vi "VI Tree.vi"   [LabVIEW 2015, in "IT8900A-E.lvlib"]
doc: "This is the instrument driver for the <INSTRUMENT NAME>. The VI Tree displays all the user-callable VIs of the instrument driver in an organized table."
uses:
  <instrlib>/IT8900/IT8900A-E.lvlib
panel:
  # "(c) 2014 <ITECH>.  ALL RIGHTS RESERVED."
  # "SEE DIAGRAM\nFOR VI TREE."
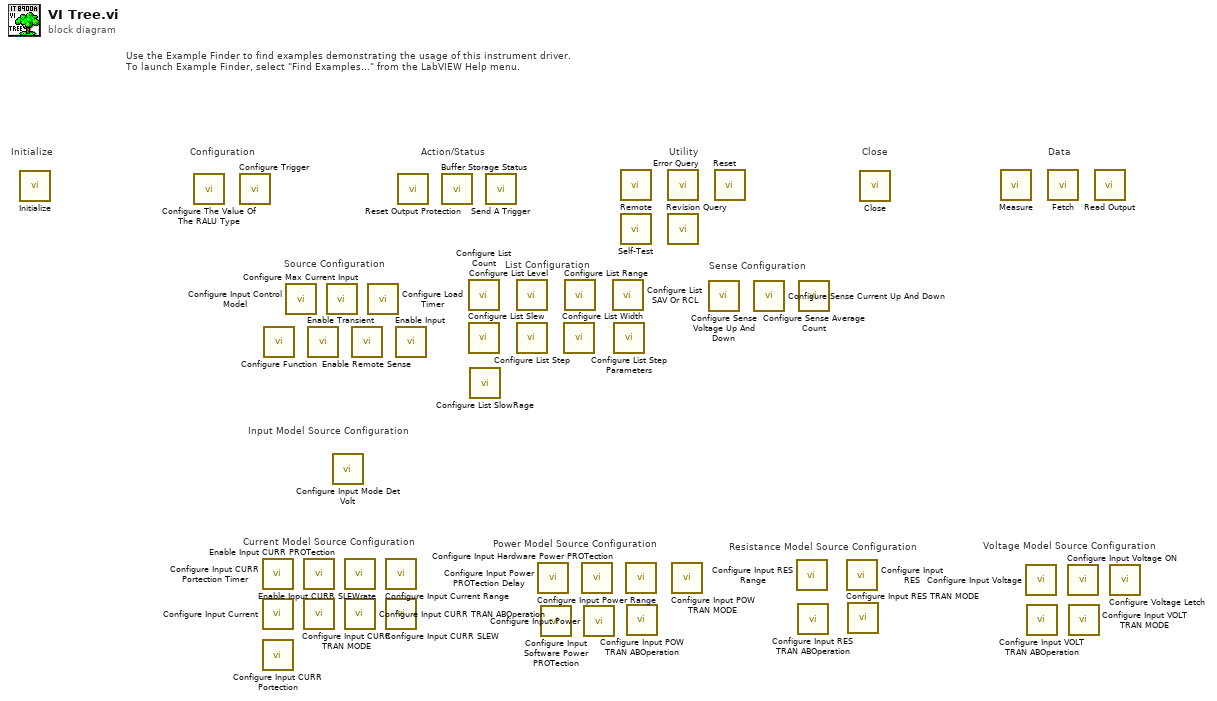
[diagram p0: block diagram]
diagram:
  # "Sense Configuration"
  # "List Configuration"
  # "Power Model Source Configuration"
  # "Resistance Model Source Configuration"
  # "Voltage Model Source Configuration"
  # "Current Model Source Configuration"
  # "Input Model Source Configuration"
  # "Source Configuration"
  # "Use the Example Finder to find examples demonstrating the usage of this instrument driver.\nTo launch Example Finder, select \"Find Examples...\" from the LabVIEW Help menu."
  # "Configuration"
  # "Utility"
  # "Data"
  # "Action/Status"
  # "Close"
  # "Initialize"
  n1 = call <instrlib>:"Initialize.vi"() -> ()  [unwired: 10 in, 2 out]
  n2 = call <instrlib>:"Configure The Value Of The RALU Type.vi"() -> ()  [unwired: 9 in, 2 out]
  n3 = call <instrlib>:"Configure Trigger.vi"() -> ()  [unwired: 10 in, 2 out]
  n4 = call <instrlib>:"Configure Input CURR Portection Timer.vi"() -> ()  [unwired: 10 in, 2 out]
  n5 = call <instrlib>:"Configure Input Current.vi"() -> ()  [unwired: 10 in, 2 out]
  n6 = call <instrlib>:"Configure Input CURR Portection.vi"() -> ()  [unwired: 10 in, 2 out]
  n7 = call <instrlib>:"Configure Function.vi"() -> ()  [unwired: 10 in, 2 out]
  n8 = call <instrlib>:"Configure Input Control Model.vi"() -> ()  [unwired: 10 in, 2 out]
  n9 = call <instrlib>:"Enable Input CURR PROTection.vi"() -> ()  [unwired: 10 in, 2 out]
  n10 = call <instrlib>:"Configure Input CURR TRAN MODE.vi"() -> ()  [unwired: 10 in, 2 out]
  n11 = call <instrlib>:"Enable Transient.vi"() -> ()  [unwired: 10 in, 2 out]
  n12 = call <instrlib>:"Configure Max Current Input.vi"() -> ()  [unwired: 10 in, 2 out]
  n13 = call <instrlib>:"Configure Input Mode Det Volt.vi"() -> ()  [unwired: 10 in, 2 out]
  n14 = call <instrlib>:"Enable Input CURR SLEWrate.vi"() -> ()  [unwired: 10 in, 2 out]
  n15 = call <instrlib>:"Configure Input CURR TRAN ABOperation.vi"() -> ()  [unwired: 10 in, 2 out]
  n16 = call <instrlib>:"Enable Remote Sense.vi"() -> ()  [unwired: 10 in, 2 out]
  n17 = call <instrlib>:"Configure Load Timer.vi"() -> ()  [unwired: 10 in, 2 out]
  n18 = call <instrlib>:"Configure Input Current Range.vi"() -> ()  [unwired: 10 in, 2 out]
  n19 = call <instrlib>:"Configure Input CURR SLEW.vi"() -> ()  [unwired: 10 in, 2 out]
  n20 = call <instrlib>:"Enable Input.vi"() -> ()  [unwired: 10 in, 2 out]
  n21 = call <instrlib>:"Reset Output Protection.vi"() -> ()  [unwired: 10 in, 2 out]
  n22 = call <instrlib>:"Buffer Storage Status.vi"() -> ()  [unwired: 7 in, 5 out]
  n23 = call <instrlib>:"Configure List Count.vi"() -> ()  [unwired: 10 in, 2 out]
  n24 = call <instrlib>:"Configure List Slew.vi"() -> ()  [unwired: 10 in, 2 out]
  n25 = call <instrlib>:"Configure List SlowRage.vi"() -> ()  [unwired: 10 in, 2 out]
  n26 = call <instrlib>:"Send A Trigger.vi"() -> ()  [unwired: 10 in, 2 out]
  n27 = call <instrlib>:"Configure List Level.vi"() -> ()  [unwired: 10 in, 2 out]
  n28 = call <instrlib>:"Configure List Step.vi"() -> ()  [unwired: 10 in, 2 out]
  n29 = call <instrlib>:"Configure Input Power PROTection Delay.vi"() -> ()  [unwired: 10 in, 2 out]
  n30 = call <instrlib>:"Configure Input Software Power PROTection.vi"() -> ()  [unwired: 10 in, 2 out]
  n31 = call <instrlib>:"Configure List Width.vi"() -> ()  [unwired: 10 in, 2 out]
  n32 = call <instrlib>:"Configure List Range.vi"() -> ()  [unwired: 10 in, 2 out]
  n33 = call <instrlib>:"Configure Input Hardware Power PROTection.vi"() -> ()  [unwired: 10 in, 2 out]
  n34 = call <instrlib>:"Configure Input Power.vi"() -> ()  [unwired: 10 in, 2 out]
  n35 = call <instrlib>:"Configure List SAV Or RCL.vi"() -> ()  [unwired: 10 in, 2 out]
  n36 = call <instrlib>:"Configure List Step Parameters.vi"() -> ()  [unwired: 10 in, 2 out]
  n37 = call <instrlib>:"Remote.vi"() -> ()  [unwired: 10 in, 2 out]
  n38 = call <instrlib>:"Self-Test.vi"() -> ()  [unwired: 8 in, 4 out]
  n39 = call <instrlib>:"Configure Input Power Range.vi"() -> ()  [unwired: 10 in, 2 out]
  n40 = call <instrlib>:"Configure Input POW TRAN ABOperation.vi"() -> ()  [unwired: 10 in, 2 out]
  n41 = call <instrlib>:"Error Query.vi"() -> ()  [unwired: 8 in, 4 out]
  n42 = call <instrlib>:"Revision Query.vi"() -> ()  [unwired: 8 in, 4 out]
  n43 = call <instrlib>:"Configure Input POW TRAN MODE.vi"() -> ()  [unwired: 10 in, 2 out]
  n44 = call <instrlib>:"Configure Sense Voltage Up And Down.vi"() -> ()  [unwired: 10 in, 2 out]
  n45 = call <instrlib>:"Reset.vi"() -> ()  [unwired: 10 in, 2 out]
  n46 = call <instrlib>:"Configure Sense Current Up And Down.vi"() -> ()  [unwired: 10 in, 2 out]
  n47 = call <instrlib>:"Configure Input RES Range.vi"() -> ()  [unwired: 10 in, 2 out]
  n48 = call <instrlib>:"Configure Input RES TRAN ABOperation.vi"() -> ()  [unwired: 10 in, 2 out]
  n49 = call <instrlib>:"Configure Sense Average Count.vi"() -> ()  [unwired: 10 in, 2 out]
  n50 = call <instrlib>:"Configure Input RES.vi"() -> ()  [unwired: 10 in, 2 out]
  n51 = call <instrlib>:"Configure Input RES TRAN MODE.vi"() -> ()  [unwired: 10 in, 2 out]
  n52 = call <instrlib>:"Close.vi"() -> ()  [unwired: 11 in, 1 out]
  n53 = call <instrlib>:"Measure.vi"() -> ()  [unwired: 9 in, 3 out]
  n54 = call <instrlib>:"Configure Input Voltage.vi"() -> ()  [unwired: 10 in, 2 out]
  n55 = call <instrlib>:"Configure Input VOLT TRAN ABOperation.vi"() -> ()  [unwired: 10 in, 2 out]
  n56 = call <instrlib>:"Fetch.vi"() -> ()  [unwired: 9 in, 3 out]
  n57 = call <instrlib>:"Configure Input Voltage ON.vi"() -> ()  [unwired: 10 in, 2 out]
  n58 = call <instrlib>:"Configure Input VOLT TRAN MODE.vi"() -> ()  [unwired: 10 in, 2 out]
  n59 = call <instrlib>:"Read Output.vi"() -> ()  [unwired: 8 in, 4 out]
  n60 = call <instrlib>:"Configure Voltage Letch.vi"() -> ()  [unwired: 10 in, 2 out]
